vi "DB_Main.vi"(8 "error in (no error)":errorcluster caption="错误输入（无错误）") -> (0 "error out":errorcluster caption="错误输出")   [LabVIEW 2016]
uses:
  <vilib>/Utility/miscctls.llb/LVRowAndColumnTypeDef.ctl
  <vilib>/Utility/miscctls.llb/LVRowAndColumnUnsignedTypeDef.ctl
  StateMachineStates.ctl
  Controls/Global.vi
panel:
  in  "刷新":bool
  in  "降序":bool
  in  "升序":bool
  in  "打印":bool
  in  "画图":bool
  in  "退出":bool
  in  "删除":bool
  in  "表格":string[][](table)
  out "XY图":cluster{"Num&Angle":dbl[], "Num&Angle":dbl[]}(graph)
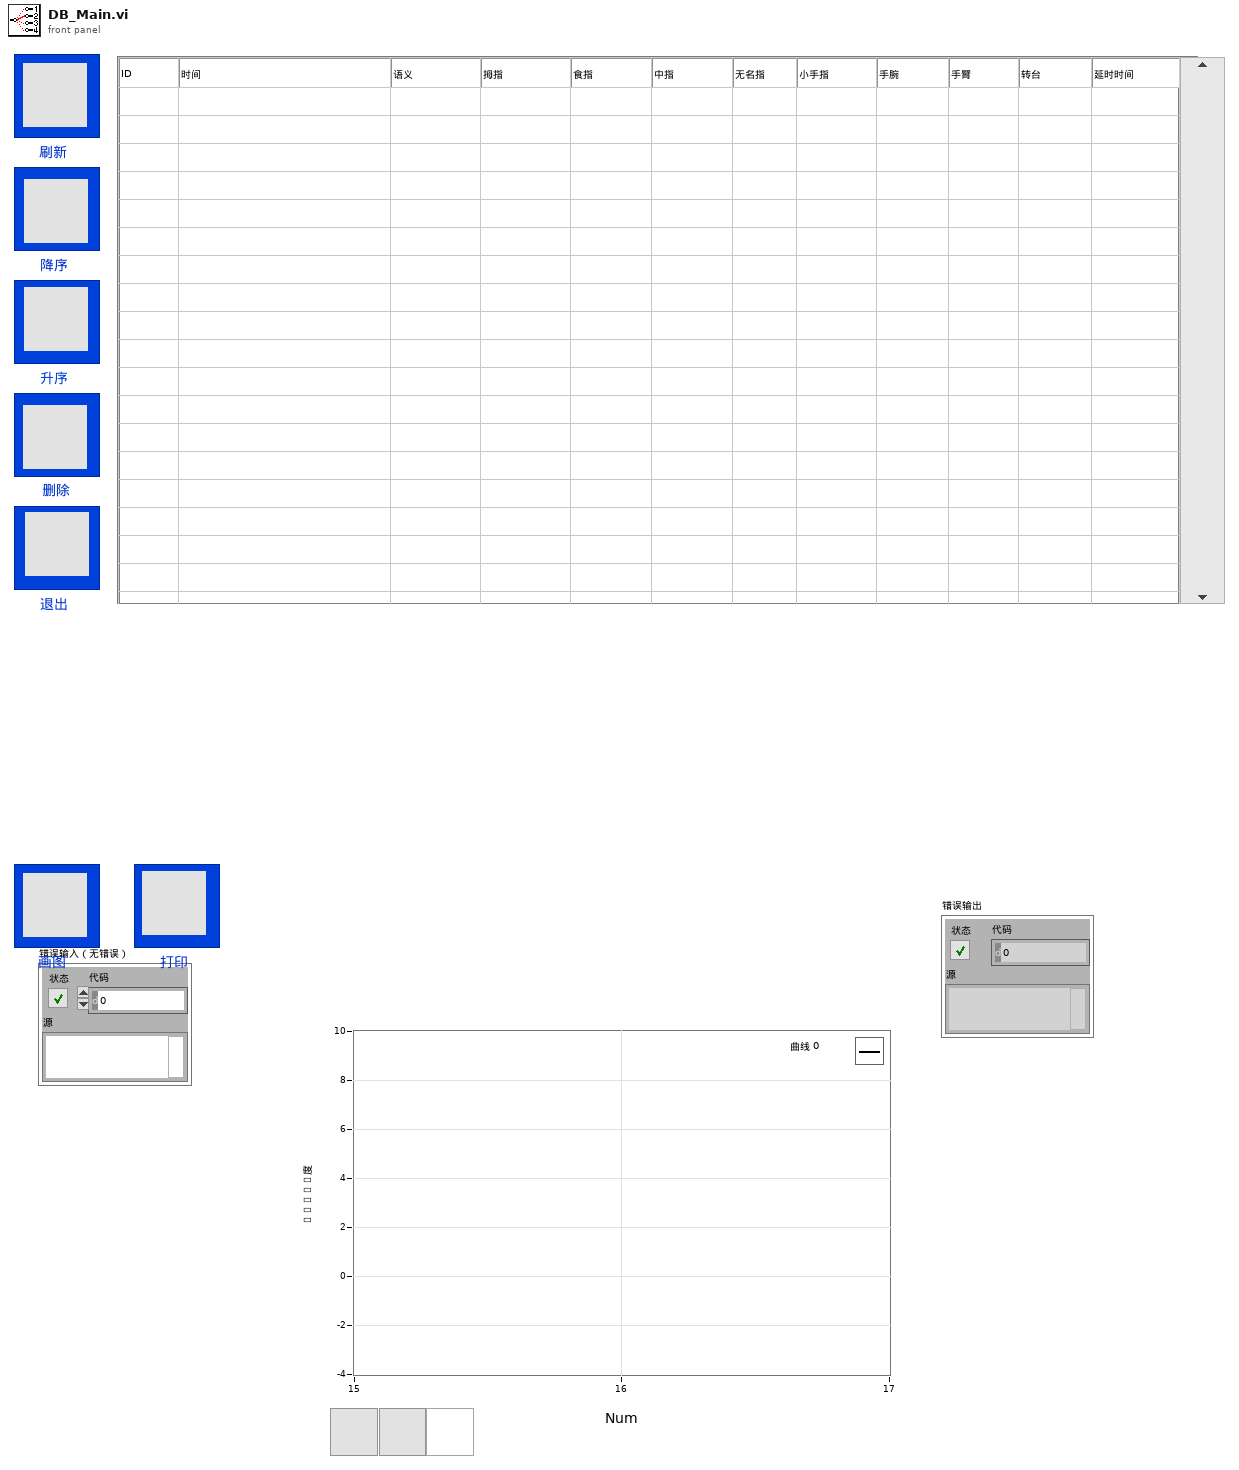
[diagram p1: front panel]
types:
  T1 = typedef "LVRowAndColumnTypeDef.ctl" = cluster{"Row":i32, "Column":i32}
  T2 = enum16{"Report", "Refresh", "Sort", "Plot", "Initialize", "Log", "Delete", "Stop", "Idle"}
  T3 = typedef "LVRowAndColumnUnsignedTypeDef.ctl" = cluster{"Row":u32, "Column":u32}
  T4 = typedef "StateMachineStates.ctl" = enum16{"Connection DB", "Creat DB", "Delete Table", "Insert DB", "Inquire Table", "Inquire All DB", "Delete All Data", "Delete Data", "Sort Data", "Inquire Last Data", ""}
  T5 = enum16{"ID", "操作者", "级数", "个数", "角度", "时间", "机匣型号", ""}
  T6 = enum16{"ID", "操作者", "级数", "个数", "角度", "时间", "机匣型号"}
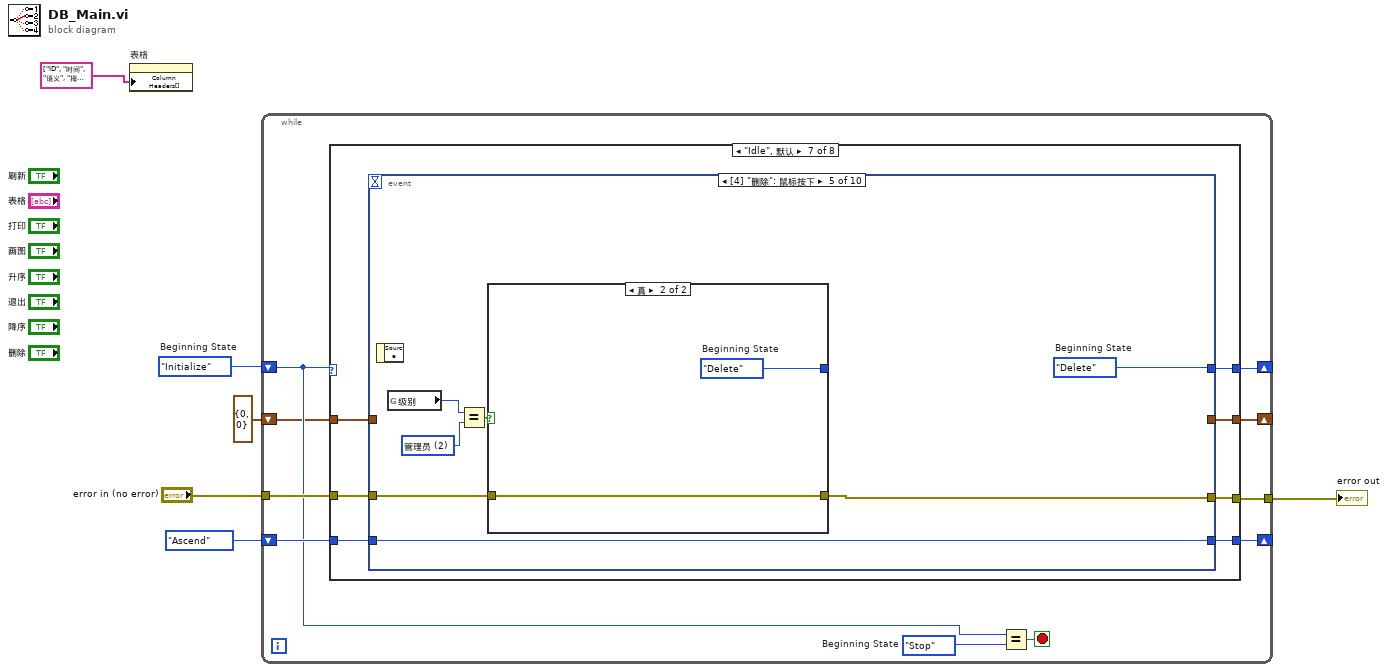
[diagram p0: block diagram]
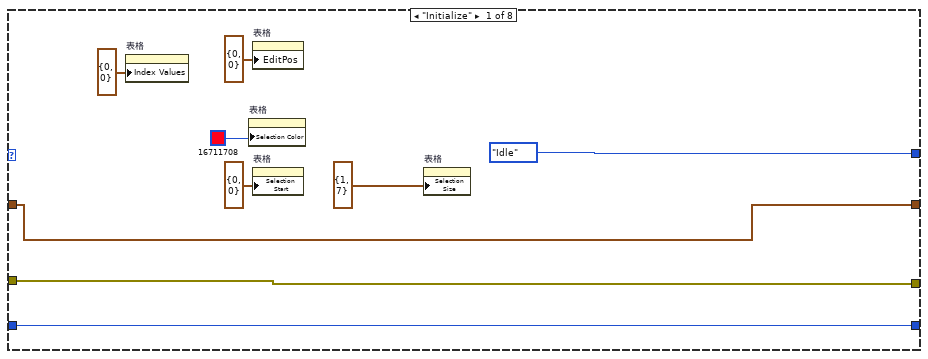
[diagram p2: hidden frame]
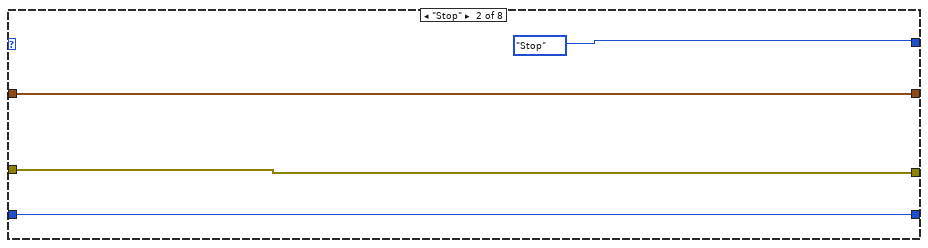
[diagram p3: hidden frame]
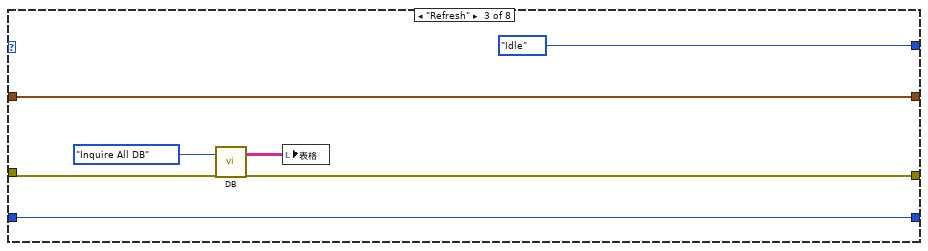
[diagram p4: hidden frame]
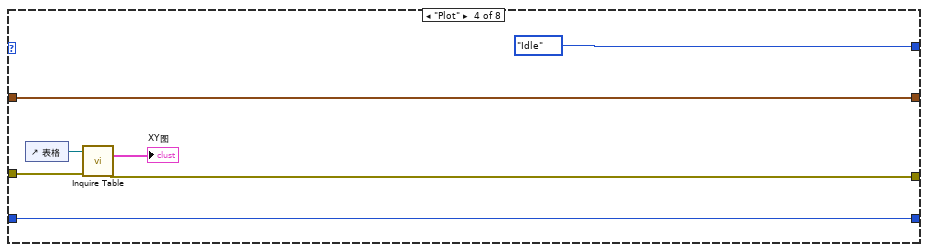
[diagram p5: hidden frame]
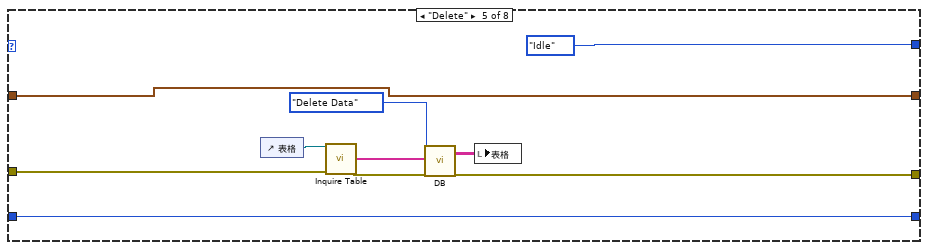
[diagram p6: hidden frame]
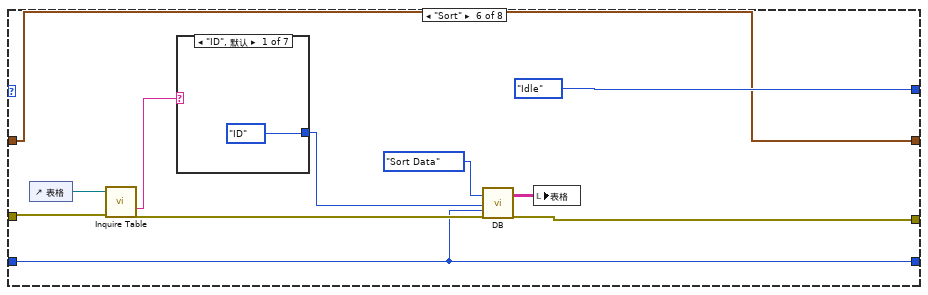
[diagram p7: hidden frame]
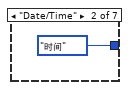
[diagram p8: hidden frame]
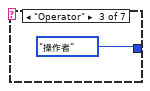
[diagram p9: hidden frame]
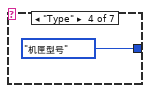
[diagram p10: hidden frame]
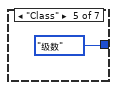
[diagram p11: hidden frame]
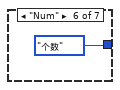
[diagram p12: hidden frame]
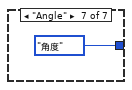
[diagram p13: hidden frame]
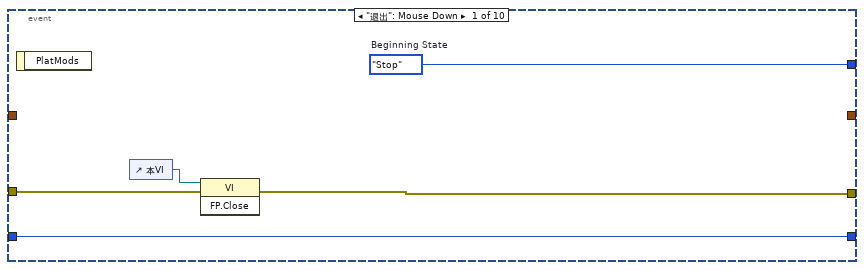
[diagram p14: hidden frame]
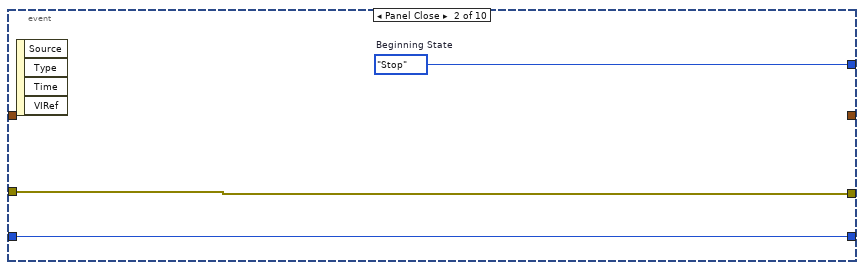
[diagram p15: hidden frame]
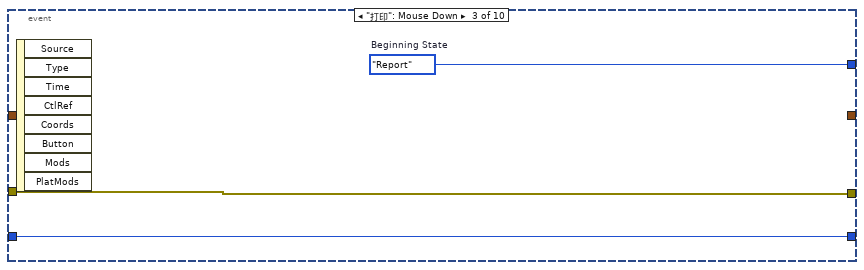
[diagram p16: hidden frame]
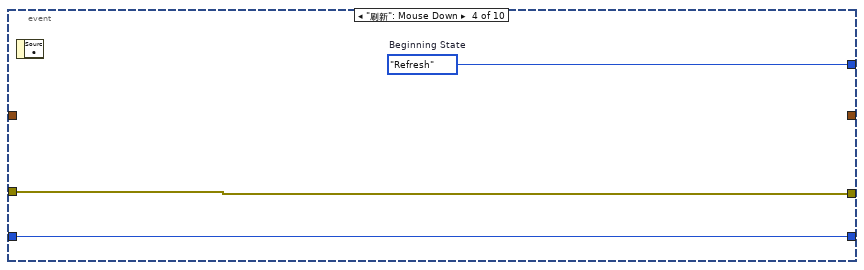
[diagram p17: hidden frame]
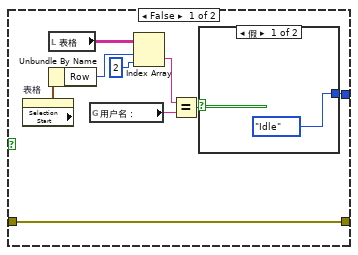
[diagram p18: hidden frame]
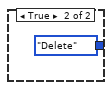
[diagram p19: hidden frame]
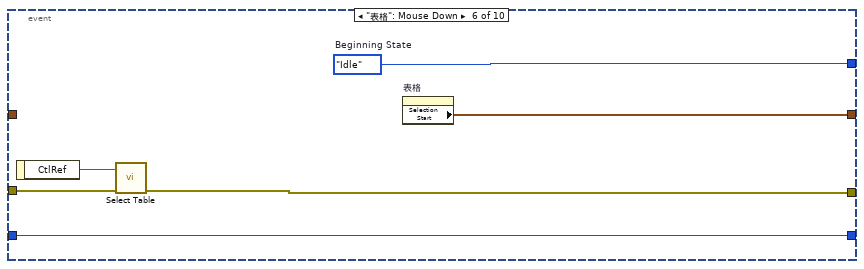
[diagram p20: hidden frame]
diagram:
  w6 = T2."Initialize"  # Beginning State
  n1 = property on="表格" class="Tbl (严格)"("Column Headers[]"=string[] ["ID", "时间", "语义", "拇指", "食指", "中指", "无名指", "小手指", "手腕", "手臂", "转台", "延时时间"] ("列首字符串[]")) -> ()  [unwired: 2 in, 2 out]
  n2 = while {
    shift-right: [w9] -> _
    shift-left: w6 -> [w11]
    tunnel: "error in (no error)" -> [w15]
    tunnel: [w14] -> w3
    shift-right: [w13] -> _
    shift-left: enum32{"Ascend", "Descend"}."Ascend" ("Order") -> [w12]
    shift-right: [w8] -> _
    shift-left: T1 {"Row"=0, "Column"=0} ("Selection Start") -> [w7]
    stop <- w16 stop-if-true
    w10 = T2."Stop"  # Beginning State
    n3 = case shown="\"Idle\", 默认" w11 {
      tunnel: w15 -> [w25 w29 w36 w41 w53 w61 w77 w169]
      tunnel: [w25 w29 w35 w40 w52 w62 w78 w169] -> w14
      tunnel: [w24 w28 w32 w43 w51 w56 w76 w170] -> w13
      tunnel: w12 -> [w24 w28 w32 w43 w51 w56 w75 w170]
      tunnel: [T2."Idle" ("Beginning State") T2."Stop" ("Beginning State") T2."Idle" ("Beginning State") T2."Idle" ("Beginning State") T2."Idle" ("Beginning State") T2."Idle" ("Beginning State") w74 w158] -> w9
      tunnel: [w17 w26 w30 w37 w44 w54 w73 w157] -> w8
      tunnel: w7 -> [w17 w26 w30 w37 w44 w54 w72 w157]
      frame "Initialize" {
        n4 = property on="表格" class="Tbl (严格)"("Index Values"=T3 {"Row"=0, "Column"=0} ("索引值")) -> ()  [unwired: 2 in, 2 out]
        n5 = property on="表格" class="Tbl (严格)"("Selection Color"=u32 16711708) -> ()  [unwired: 2 in, 2 out]
        n6 = property on="表格" class="Tbl (严格)"("EditPos"=T1 {"Row"=0, "Column"=0} ("编辑位置")) -> ()  [unwired: 2 in, 2 out]
        n7 = property on="表格" class="Tbl (严格)"("Selection Start"=T1 {"Row"=0, "Column"=0} ("选择区域起始")) -> ()  [unwired: 2 in, 2 out]
        n8 = property on="表格" class="Tbl (严格)"("Selection Size"=T1 {"Row"=1, "Column"=7} ("选择区域大小")) -> ()  [unwired: 2 in, 2 out]
      }
      frame "Stop" {
      }
      frame "Refresh" {
        n9 = call "DB.vi"("Beginning State"=StateMachineStates."Inquire All DB", "ErrI(No Error)"=w36) -> ("Item Data"=w33:string[][], "ErrO"=w35:errorcluster)  [unwired: 11 in, 5 out]
        n10 = local write "表格"(w33) -> ()
      }
      frame "Plot" {
        n11 = control-ref of="表格"() -> (w42:refnum<vi>)
        n12 = call "Inquire Table.vi"("表格"=w42, "error in (no error)"=w41) -> ("XY图/Num&Angle"=→"XY图":cluster{dbl[], dbl[]}, "error out"=w40:errorcluster)  [unwired: 7 in, 5 out]
      }
      frame "Delete" {
        n13 = control-ref of="表格"() -> (w45:refnum<vi>)
        n14 = call "Inquire Table.vi"("表格"=w45, "error in (no error)"=w53) -> ("选择的ID"=w49:string[], "error out"=w48:errorcluster)  [unwired: 7 in, 5 out]
        n15 = call "DB.vi"("Beginning State"=StateMachineStates."Delete Data", "Delete Num"=w49, "ErrI(No Error)"=w48) -> ("Item Data"=w46:string[][], "ErrO"=w52:errorcluster)  [unwired: 10 in, 5 out]
        n16 = local write "表格"(w46) -> ()
      }
      frame "Sort" {
        n17 = control-ref of="表格"() -> (w60:refnum<vi>)
        n18 = call "Inquire Table.vi"("表格"=w60, "error in (no error)"=w61) -> ("选择的列首"=w59:string, "error out"=w64:errorcluster)  [unwired: 7 in, 5 out]
        n19 = case shown="\"ID\", 默认" w59 {
          tunnel: [T5."ID" ("Sort As") enum16{"ID", "操作者", "级数", "个数", "角度", "时间"}."时间" ("Sort As") enum16{"ID", "操作者", "级数", "个数", "角度", "时间"}."操作者" ("Sort As") T6."机匣型号" ("Sort As") enum16{"ID", "操作者", "级数", "个数", "角度", "时间"}."级数" ("Sort As") enum16{"ID", "操作者", "级数", "个数", "角度", "时间"}."个数" ("Sort As") enum16{"ID", "操作者", "级数", "个数", "角度", "时间"}."角度" ("Sort As")] -> w58
          frame "ID", Default {
          }
          frame "Date/Time" {
          }
          frame "Operator" {
          }
          frame "Type" {
          }
          frame "Class" {
          }
          frame "Num" {
          }
          frame "Angle" {
          }
        }
        n20 = call "DB.vi"("Beginning State"=StateMachineStates."Sort Data", "Sort As"=w58, "Order"=w56, "ErrI(No Error)"=w64) -> ("Item Data"=w57:string[][], "ErrO"=w62:errorcluster)  [unwired: 9 in, 5 out]
        n21 = local write "表格"(w57) -> ()
      }
      frame "Idle", Default {
        n22 = event shown="[4] \"删除\": 鼠标按下" {
          selector: _ -> [_ _ _ _ _ _ _ _ _ _]
          dyn-events: _ -> [_ _ _ _ _ _ _ _ _ _]
          timeout: _ -> [_ _ _ _ _ _ _ _ _ _]
          tunnel: [w79 w84 w87 w90 w93 w114 T2."Idle" ("Beginning State") w149 w152 w154] -> w74
          tunnel: [w80 w85 w89 w92 w95 w116 w130 w151 _ w155] -> w78
          tunnel: w77 -> [w81 w85 w89 w92 w94 w117 w130 w151 _ w155]
          tunnel: [w83 w86 w88 w91 w99 w118 w129 enum32{"Ascend", "Descend"}."Ascend" ("Order") enum32{"Ascend", "Descend"}."Descend" ("Order") w156] -> w76
          tunnel: w75 -> [w83 w86 w88 w91 w99 w118 w129 _ _ w156]
          tunnel: [_ _ _ _ _ w113 _ _ _ _] -> w73
          tunnel: w72 -> [_ _ _ _ _ _ _ _ _ _]
          event "退出": Mouse Down {
            w79 = T2."Stop"  # Beginning State
            n23 = event-data() -> ()  [unwired: 1 in, 1 out]
            n24 = control-ref of="本VI"() -> (w82:refnum<vi>)
            n25 = invoke class="VI" method="FP.Close"(reference=w82, error in=w81) -> (error out=w80:errorcluster)  [unwired: 1 in, 2 out]
          }
          event Panel Close {
            w84 = T2."Stop"  # Beginning State
            n26 = event-data() -> ()  [unwired: 1 in, 4 out]
          }
          event "打印": Mouse Down {
            w87 = T2."Report"  # Beginning State
            n27 = event-data() -> ()  [unwired: 1 in, 8 out]
          }
          event "刷新": Mouse Down {
            w90 = T2."Refresh"  # Beginning State
            n28 = event-data() -> ()  [unwired: 1 in, 1 out]
          }
          event "删除": Mouse Down {
            w93 = T2."Delete"  # Beginning State
            w97 = u16 2 items=["其他", "普通用户", "管理员"] ("级别")
            n29 = event-data() -> ()  [unwired: 1 in, 1 out]
            n30 = global read "Global.vi" "级别"() -> (w98:u16)
            n31 = Equal?(x=w98, y=w97) -> (x = y?=w96:bool)
            n32 = case shown="真" w96 {
              tunnel: [w100 w112] -> _
              tunnel: [w108 w111] -> w95
              tunnel: w94 -> [w108 w111]
              frame False {
                n33 = property on="表格" class="Tbl (严格)"() -> ("Selection Start"=w106:T1)  [unwired: 2 in, 2 out]
                n34 = local read "表格"() -> (w107:string[][])
                n35 = Unbundle By Name(w106) -> ("Row"=w105:i32)
                n36 = global read "Global.vi" "用户名："() -> (w102:string)
                n37 = Index Array(array=w107, index (row)=w105, index (col)=2 ("disabled index (col)")) -> (element=w103:string)
                n38 = Equal?(x=w103, y=w102) -> (x = y?=w101:bool)
                n39 = case shown="假" w101 {
                  tunnel: [T2."Idle" ("f") T2."Delete" ("Beginning State")] -> w100
                  frame False {
                  }
                  frame True {
                  }
                }
              }
              frame True {
                w112 = T2."Delete"  # Beginning State
              }
            }
          }
          event "表格": Mouse Down {
            w114 = T2."Idle"  # Beginning State
            n40 = event-data() -> ("CtlRef"=w115:refnum<vi>)  [unwired: 1 in]
            n41 = call "Select Table.vi"("error in (no error)"=w117, "表格"=w115) -> ("error out"=w116:errorcluster)  [unwired: 9 in]
            n42 = property on="表格" class="Tbl (严格)"() -> ("Selection Start"=w113:T1)  [unwired: 2 in, 2 out]
          }
          event "表格": Value Change {
            n43 = event-data() -> ("OldVal"=w126:string[][], "NewVal"=w125:string[][], "OldVal"=w124:string[][])  [unwired: 1 in]
            n44 = property on="表格" class="Tbl (严格)"() -> ("Selection Start"=w127:T1)  [unwired: 2 in, 2 out]
            n45 = Unbundle By Name(w127) -> ("Row"=w119:i32)
            n46 = Index Array(array=w125, index (row)=w119) -> (element=w123:string[])  [unwired: 1 in]
            n47 = Index Array(array=w124, index (row)=w119) -> (element=w122:string[])  [unwired: 1 in]
            n48 = Equal?(x=w123, y=w122) -> (x = y?=w121:bool[])
            n49 = And Array Elements(Boolean array=w121) -> (logical AND=w120:bool)
            n50 = case shown="真" w120 {
              tunnel: w126 -> [w139 _]
              tunnel: w119 -> [w143 _]
              tunnel: w123 -> [w142 _]
              tunnel: w119 -> [w132 _]
              frame False {
                n51 = Index Array(array=w142, index=0) -> (element=w140:string)
                n52 = Index Array(array=w139, index (col)=0 ("disabled index (col)")) -> (element=w134:string[])  [unwired: 1 in]
                n53 = Delete From Array(array=w134, length=1, index=w132) -> (array with subset deleted=w131:string[])  [unwired: 1 out]
                n54 = Search 1D Array(1D array=w131, element=w140) -> (index of element=w138:i32)  [unwired: 1 in]
                n55 = Equal?(x=-1, y=w138) -> (x = y?=w136:bool)
                n56 = case shown="真" w136 {
                  tunnel: w143 -> [_ _]
                  tunnel: w142 -> [_ _]
                  tunnel: w139 -> [_ w146]
                  frame False {
                    n57 = call "DB.vi"("Beginning State"=StateMachineStates."Inquire All DB") -> ("Item Data"=w144:string[][])  [unwired: 12 in, 6 out]
                    n58 = local write "表格"(w144) -> ()
                  }
                  frame True {
                    n59 = local write "表格"(w146) -> ()
                  }
                }
              }
              frame True {
                n60 = call "DB.vi"("Beginning State"=StateMachineStates."Inquire All DB") -> ("Item Data"=w147:string[][])  [unwired: 12 in, 6 out]
                n61 = local write "表格"(w147) -> ()
              }
            }
          }
          event "升序": Mouse Down {
            w149 = T2."Sort"  # Beginning State
            n62 = event-data() -> ()  [unwired: 1 in, 1 out]
          }
          event "降序": Value Change {
            w152 = T2."Sort"  # Beginning State
            n63 = event-data() -> ()  [unwired: 1 in, 1 out]
          }
          event "画图": Mouse Down {
            w154 = T2."Plot"  # Beginning State
            n64 = event-data() -> ()  [unwired: 1 in, 1 out]
          }
        }
      }
      frame "Report" {
        w158 = T2."Idle"  # Beginning State
        n65 = control-ref of="表格"() -> (w168:refnum<vi>)
        n66 = Get Date/Time String() -> (date string=w164:string, time string=w165:string)  [unwired: 3 in]
        n67 = global read "Global.vi" "Grade"() -> (w159:string)
        n68 = call "Inquire Table.vi"("表格"=w168) -> ("Type"=w162:string, "Class&Num&Angle"=w167:dbl[][], "error out"=w166:errorcluster)  [unwired: 8 in, 4 out]
        n69 = Concatenate Strings(w164, "-" ("字符串"), w165) -> (w163:string)
        n70 = global read "Global.vi" "用户名："() -> (w160:string)
        n71 = call "WordRp.vi"("Type"=w162, "Date"=w163, "Grade"=w159, "data"=w167, "error in (no error)"=w166, "Operator"=w160) -> ()  [unwired: 12 in, 2 out]
      }
    }
    n72 = Equal?(x=w11, y=w10) -> (x = y?=w16:bool)
  }
  "error out" <- w3
